vi "Find Buffer Index.vi"(9 "buffer id":string, 11 "Session Transaction Buffers":T1[](array[typedef])) -> (2 "index":i32)   [LabVIEW 2015, in "RelayInterface.lvclass"]
uses:
  RelayInterface.lvclass
  Session Transaction Buffer.ctl
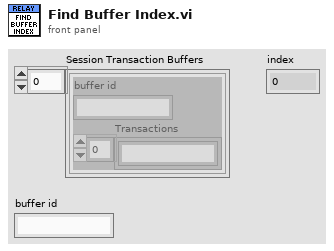
[diagram p1: front panel]
types:
  T1 = typedef "RelayInterface.lvclass/Session Transaction Buffer.ctl" = cluster{"buffer id":string, "Transactions":string[]}
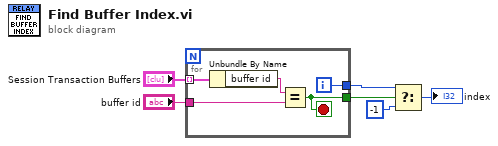
[diagram p0: block diagram]
diagram:
  n1 = for {
    tunnel: "Session Transaction Buffers" -> [w11] mode=indexing
    tunnel: "buffer id" -> [w9]
    tunnel: [w7] -> w4
    tunnel: [w8] -> w3
    i -> [w8]
    stop <- w7 stop-if-true
    n2 = Unbundle By Name(w11) -> ("buffer id"=w10:string)
    n3 = Equal?(x=w10, y=w9) -> (x = y?=w7:bool)
  }
  n4 = Select(t=w3, s=w4, f=-1) -> (s? t:f=→"index":i32)
